vi "MEI.vi"(6 "Numero Stadi":dbl, 7 "TIPO POMPA":u16(ring)=3 items=["ESOB (1450)", "ESOB (2900)", "ESCC (1450)", "ESCC (2900)", "ESCCi (1450)", "ESCCi (2900)", "MS-V (2900)", "MSS (2900)"], 10 "INDEX":T1, 11 "Curva":string[][](array[string])) -> (0 "TIPO POMPA 2":u16(ring)=3 items=["ESOB (1450)", "ESOB (2900)", "ESCC (1450)", "ESCC (2900)", "ESCCi (1450)", "ESCCi (2900)", "MS-V (2900)", "MSS (2900)"], 1 "Numero Stadi 2":dbl, 2 "MEI":string, 3 "colonna mei":string[](array[string]), 5 "annulla ?":bool)   [LabVIEW 2016]
uses:
  TypeDef/Indici.ctl
  <vilib>/Analysis/6fits.llb/Curve Fitting Criteria.ctl
  <vilib>/Analysis/polynomials.llb/nth Derivative of Polynomial (DBL).vi
  <vilib>/Analysis/polynomials.llb/Polynomial Roots (DBL).vi
  <vilib>/Analysis/polynomials.llb/Polynomial Plot (Range).vi
  <vilib>/Analysis/polynomials.llb/Scalar Polynomial Evaluation (DBL).vi
  <vilib>/Analysis/NI_AALPro.lvlib
panel:
  in  "annulla":bool
  out "NewVal":u16
  in  "reinizializza tabella":bool
  in  "elimina acq":bool
  out "Q_PL [l/min]":dbl
  out "Q_OL [l/min]":dbl
  out "Q_BEP [l/min]":dbl
  out "R-square 2":dbl caption="R-square"
  out "R-square":dbl
  in  "AUTOSCALA Q-H":bool=TRUE
  in  "AUTOSCALA Q-ETA":bool=TRUE
  in  "OK Button":bool
  in  "polynomial order Q-H":i32=4
  in  "polynomial order Q-Etap":i32=4
  in  "Test data":i32(listbox)
  out "indice":i32
  out "C_MEI":dbl
  out "C_OL":dbl
  out "C_PL":dbl
  out "C_BEP":dbl
  out "F_Eta":dbl
  out "n_S":dbl
  out "Velocità Nominale":dbl
  out "H_BEP [m]":dbl
  out "Q-H":cluster{"Ramp Pattern":dbl[], "P(A)":dbl[]}[](graph)
  out "ETA_PL [%]":dbl
  out "ETA_OL [%]":dbl
  out "Q_PL [m3/h]":dbl
  out "Q_OL [m3/h]":dbl
  out "ETA_BEP [%]":dbl
  out "Q-ETAp":cluster{"Ramp Pattern":dbl[], "P(A)":dbl[]}[](graph)
  out "Q_BEP [m3/h]":dbl
  # "CALCOLO INDICE MEI"
  # "Selezionare tipologia pompa e numero stadi"
  # "Seleziona ordine delle polinomiali"
  # "Risultati calcoli intermedi"
  # "RISULTATO"
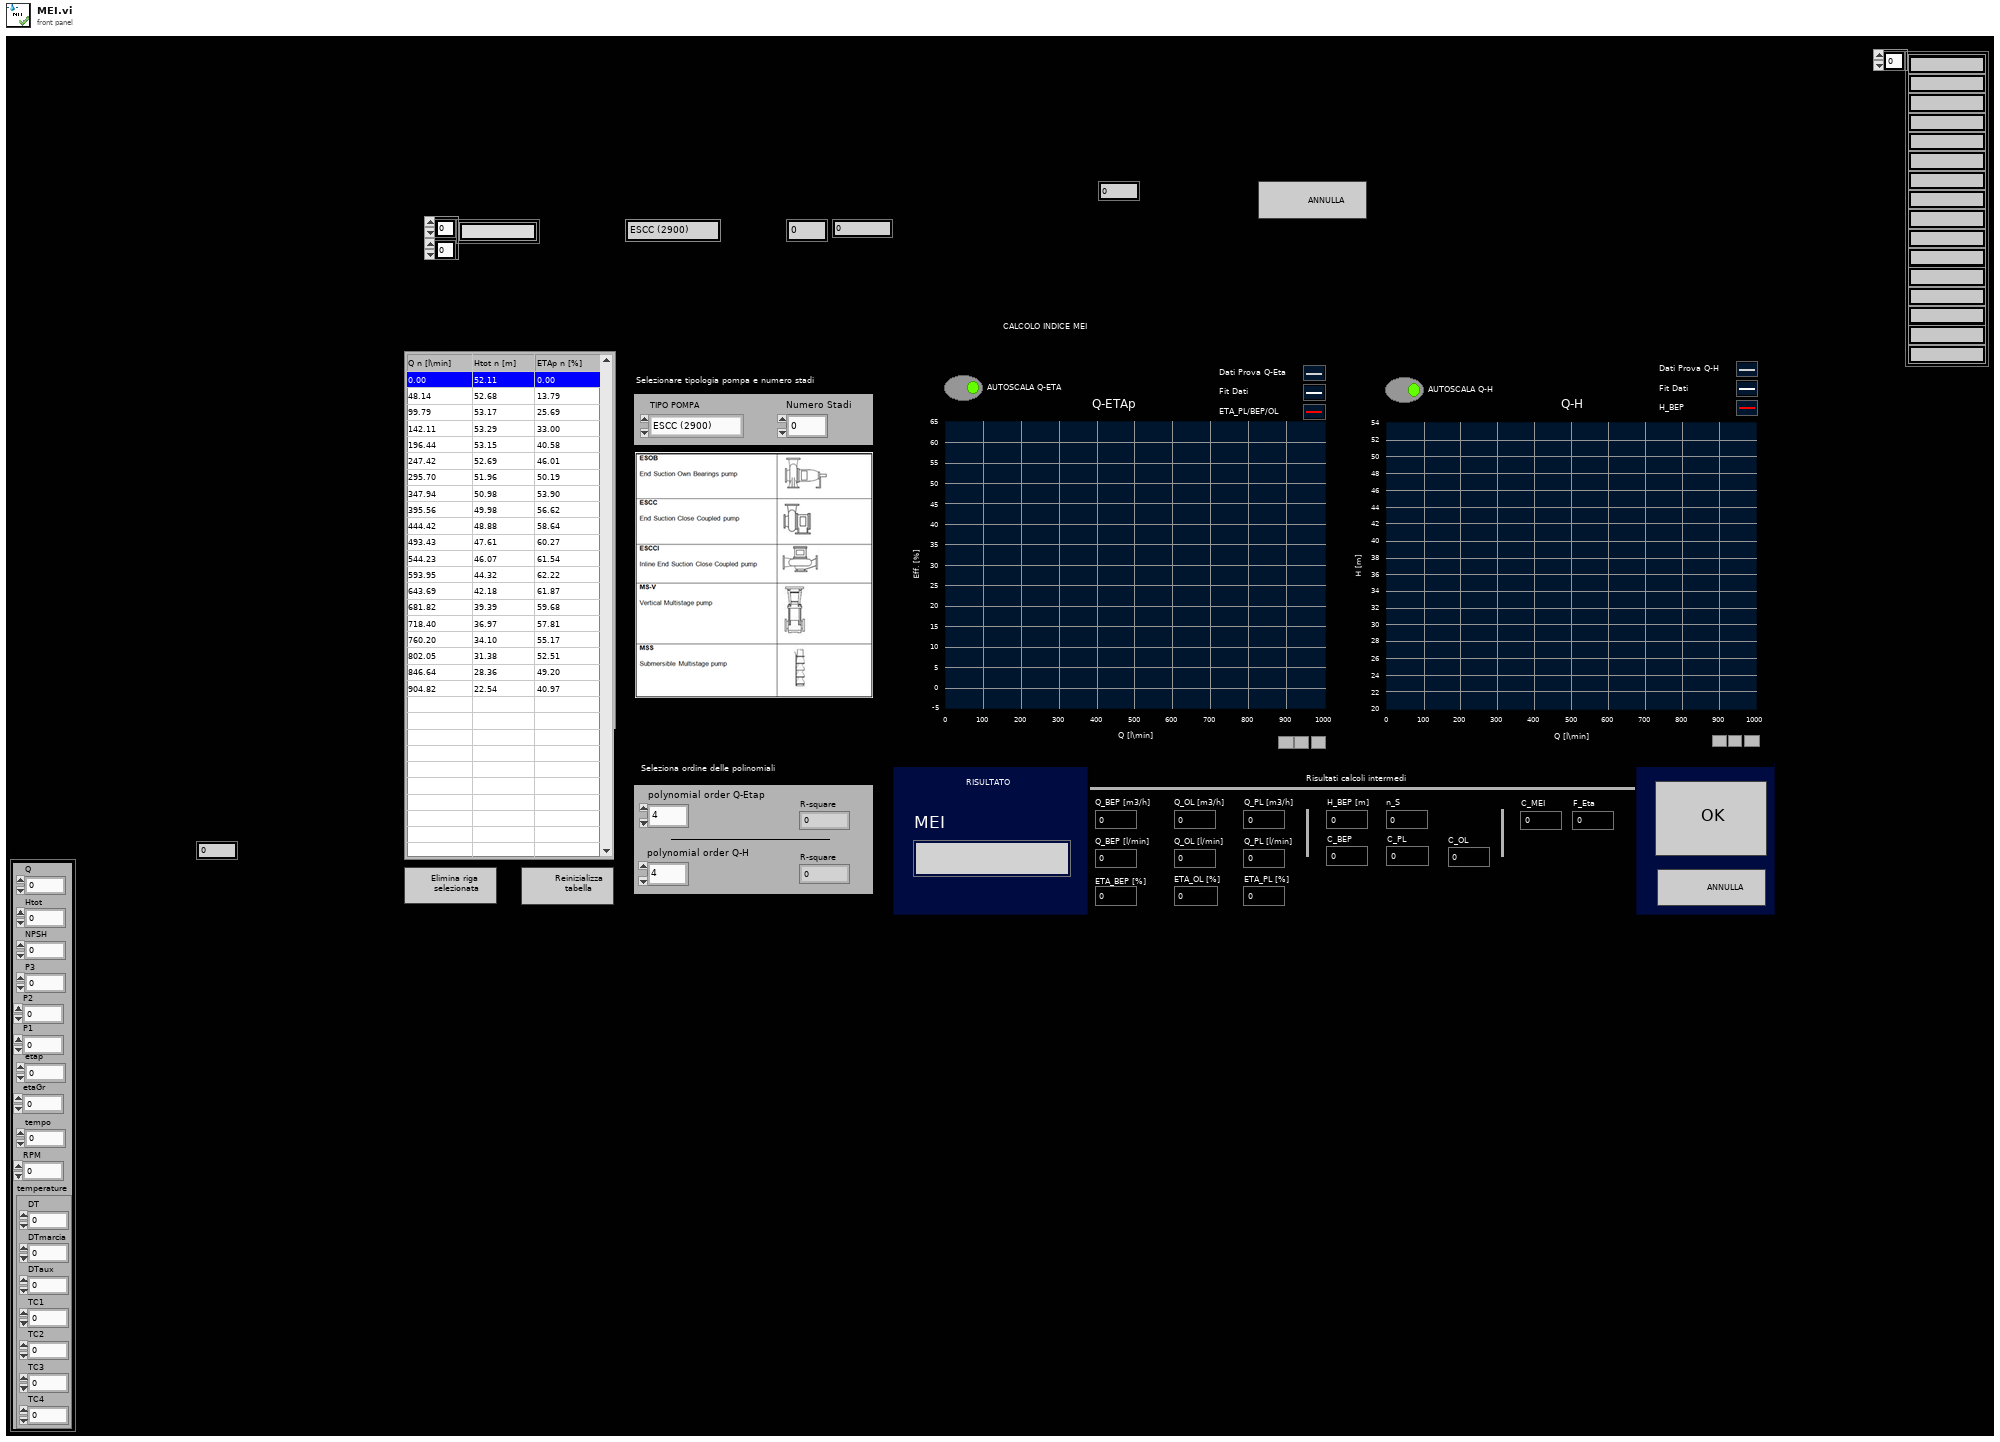
[diagram p1: front panel]
types:
  T1 = typedef "Indici.ctl" = cluster{"Q":i32, "Htot":i32, "NPSH":i32, "P3":i32, "etap":i32, "temperature":cluster{"DT":i32, "DTmarcia":i32, "DTaux":i32, "TC1":i32, "TC2":i32, "TC3":i32, "TC4":i32}, "tempo":i32, "P2":i32, "P1":i32, "etaGr":i32, "RPM":i32}
  T2 = typedef "NI_AALPro.lvlib/Curve Fitting Criteria.ctl" = u16
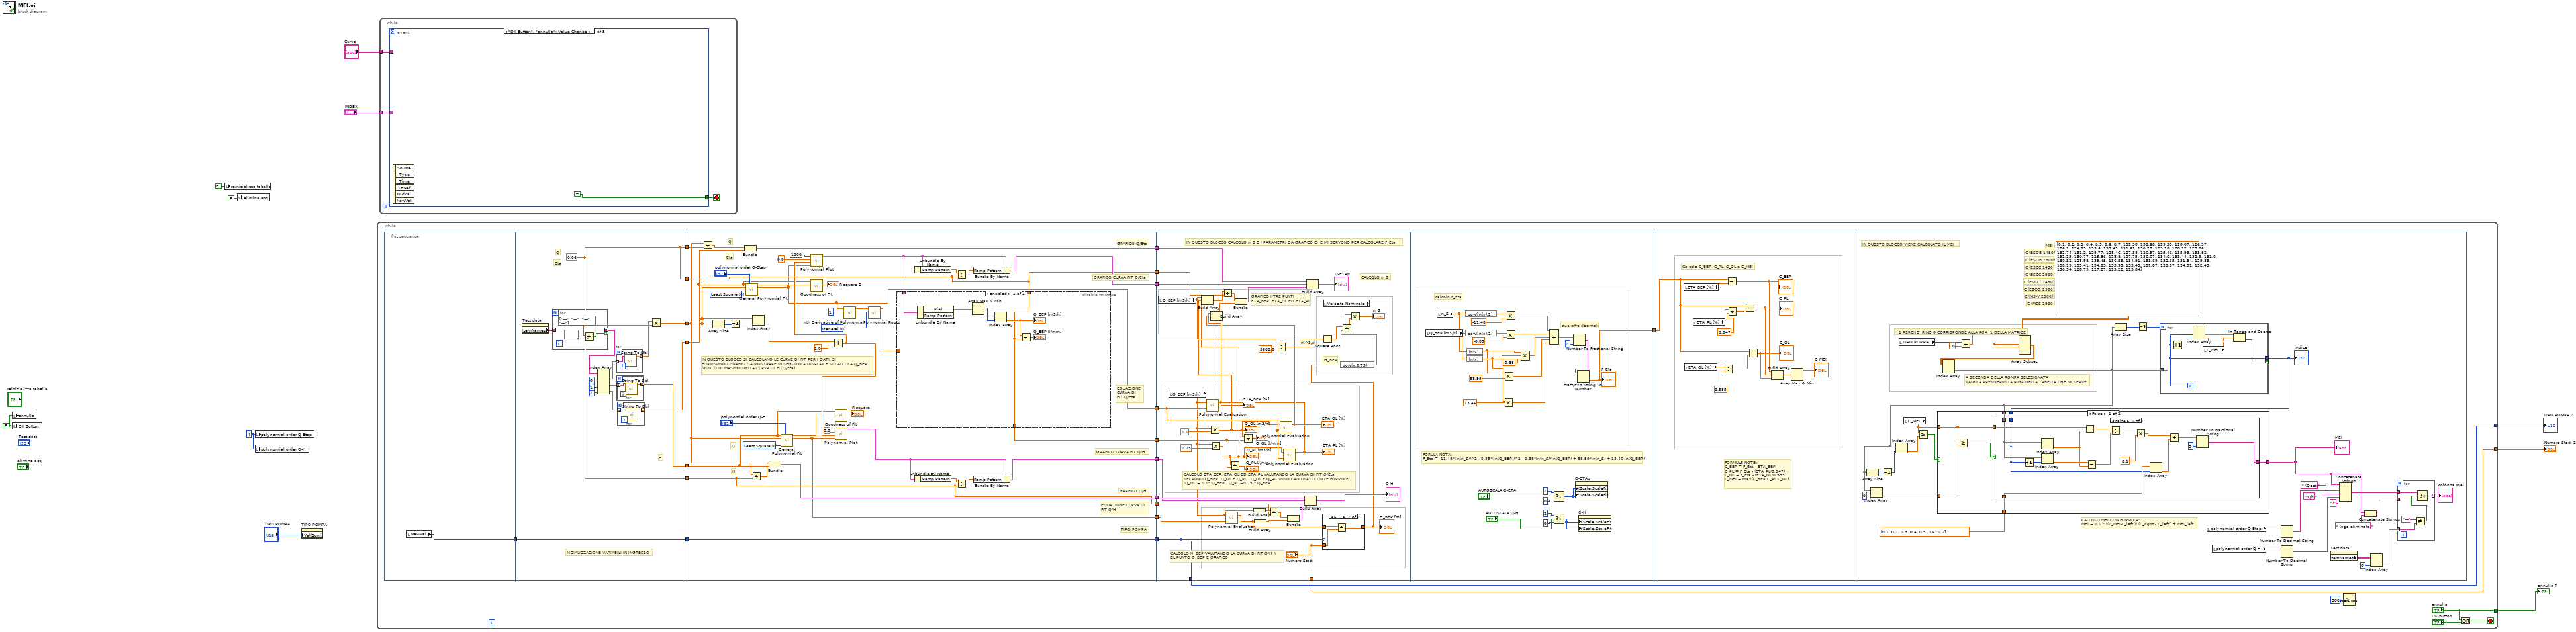
[diagram p0: block diagram]
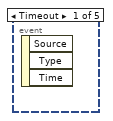
[diagram p2: hidden frame]
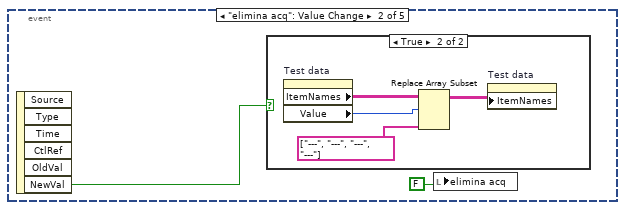
[diagram p3: hidden frame]
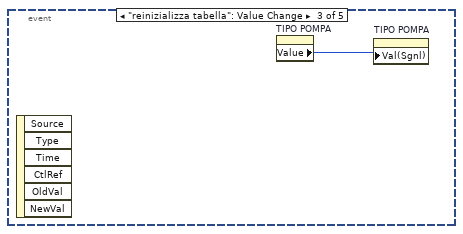
[diagram p5: hidden frame]
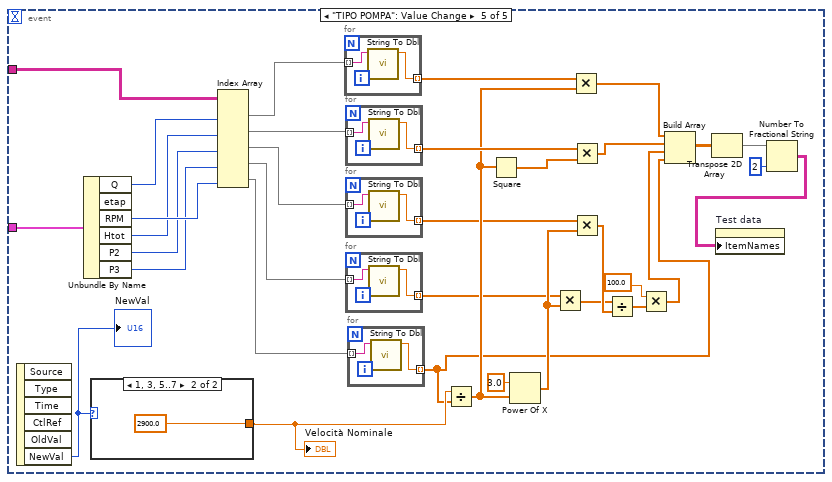
[diagram p6: hidden frame]
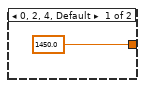
[diagram p7: hidden frame]
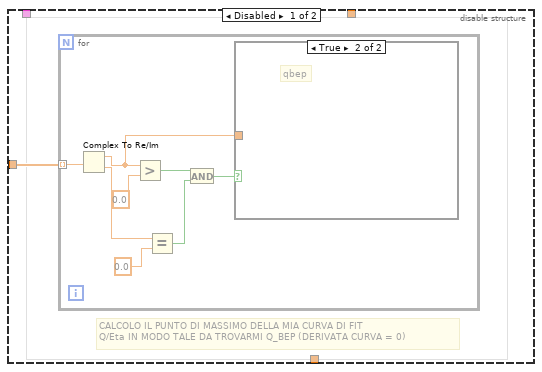
[diagram p8: hidden frame]
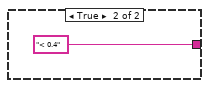
[diagram p11: hidden frame]
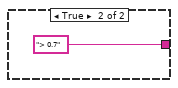
[diagram p12: hidden frame]
diagram:
  w1 = 4 ("polynomial order Q-Etap")
  w3 = FALSE ("OK Button")
  n1 = local write "annulla"(w3) -> ()
  n2 = local write "OK Button"(w3) -> ()
  n3 = local write "reinizializza tabella"(FALSE ("reinizializza tabella")) -> ()
  n4 = local write "elimina acq"(FALSE ("elimina acq")) -> ()
  n5 = local write "polynomial order Q-Etap"(w1) -> ()
  n6 = local write "polynomial order Q-H"(w1) -> ()
  n7 = property on="TIPO POMPA" class="Ring (strict)"("Val(Sgnl)"="TIPO POMPA") -> ()  [unwired: 2 in, 2 out]
  n8 = while {
    tunnel: [w22] -> w10
    tunnel: [w21] -> w9
    tunnel: ["annulla"] -> w2
    stop <- w12 stop-if-true
    n9 = flat-sequence {
      tunnel: [w36] -> w13
      tunnel: [w50] -> w35
      tunnel: [w42] -> w34
      tunnel: [w37] -> w33
      tunnel: [w49] -> w20
      tunnel: [w49] -> w19
      tunnel: [w49] -> w18
      tunnel: [w40] -> w14
      tunnel: w13 -> [w37]
      tunnel: [w93] -> w32
      tunnel: [w67] -> w31
      tunnel: [w75] -> w30
      tunnel: [w92] -> w29
      tunnel: [w63] -> w28
      tunnel: [w88] -> w27
      tunnel: w35 -> [w72]
      tunnel: w34 -> [w80]
      tunnel: [w87] -> w26
      tunnel: w33 -> [w87]
      tunnel: w20 -> [w73]
      tunnel: w19 -> [w62]
      tunnel: w18 -> [w61]
      tunnel: [w61] -> w17
      tunnel: [w62] -> w16
      tunnel: [w60] -> w15
      tunnel: w14 -> [w77]
      tunnel: w32 -> [w139]
      tunnel: w31 -> [w138]
      tunnel: w30 -> [w155]
      tunnel: w29 -> [w153]
      tunnel: w28 -> [w152]
      tunnel: w27 -> [w147]
      tunnel: w26 -> [w132]
      tunnel: [w132] -> w22
      tunnel: ["Numero Stadi"] -> w21
      tunnel: w17 -> [w128]
      tunnel: w16 -> [w125]
      tunnel: w15 -> [w121]
      tunnel: [w187] -> w25
      tunnel: w25 -> [w198]
      frame #0 {
        n10 = local read "NewVal"() -> (w36:u16)
      }
      frame #1 {
        w49 = 0.06
        # "NIZIALIZZAZIONE VARIABILI IN INGRESSO"
        # "Eta"
        # "H"
        # "Q"
        n11 = property on="Test data" class="MCListbox (strict)"() -> ("ItemNames"=w39:string[][])  [unwired: 2 in, 2 out]
        n12 = for {
          tunnel: w39 -> [w52] mode=indexing
          tunnel: [w52] -> w38 mode=indexing if=w51
          n13 = Not Equal?(x=string[] ["---", "---", "---", "---"] ("new element/subarray"), y=w52) -> (x != y?=w51:bool)
        }
        n14 = Index Array(array=w38, index (col) #1=0 ("disabled index (col)"), index (col) #2=1 ("index (col)"), index (col) #3=2 ("index (col)")) -> (element #1=w45:string[], element #2=w43:string[], element #3=w41:string[])  [unwired: 3 in]
        n15 = for {
          tunnel: w45 -> [w59] mode=indexing
          tunnel: [w58] -> w44 mode=indexing
          n16 = call "String To Dbl.vi"("String"=w59) -> ("Numeric"=w58:dbl)  [unwired: 10 in]
        }
        n17 = for {
          tunnel: w43 -> [w57] mode=indexing
          tunnel: [w56] -> w42 mode=indexing
          n18 = call "String To Dbl.vi"("String"=w57) -> ("Numeric"=w56:dbl)  [unwired: 10 in]
        }
        n19 = for {
          tunnel: w41 -> [w55] mode=indexing
          tunnel: [w54] -> w40 mode=indexing
          n20 = call "String To Dbl.vi"("String"=w55) -> ("Numeric"=w54:dbl)  [unwired: 10 in]
        }
        n21 = Multiply(x=w44, y=w49) -> (x*y=w50:dbl[])
      }
      frame #2 {
        w90 = T2 0 items=["Least Square", "Least Absolute Residual", "Bisquare"] ("method")
        w97 = u16 0 items=["General", "Simple Classification", "Refinement", "Advanced Refinement"] ("option")
        w101 = T2 0 items=["Least Square", "Least Absolute Residual", "Bisquare"] ("method")
        # "TIPO POMPA"
        # "IN QUESTO BLOCCO SI CALCOLANO LE CURVE DI FIT PER I DATI, SI \nFORNISONO I GRAFICI DA MOSTRARE IN SEGUITO A DISPLAY E SI CALCOLA Q_BEP \n(PUNTO DI MASIMO DELLA CURVA DI FITQ/Eta)"
        # "H"
        # "Q"
        # "EQUAZIONE CURVA DI \nFIT Q/H"
        # "EQUAZIONE \nCURVA DI \nFIT Q/Eta"
        # "GRAFICO CURVA FIT Q/H"
        # "GRAFICO Q/H"
        # "GRAFICO CURVA FIT Q/Eta"
        # "GRAFICO Q/Eta"
        # "Q"
        # "Eta"
        n22 = Divide(x=w72, y=w73) -> (x/y=w74:dbl[])
        n23 = Array Size(array=w72) -> (size(s)=w86:i32)
        n24 = Decrement(x=w86) -> (x-1=w85:i32)
        n25 = Bundle(w74, w77) -> (w93:cluster{dbl[], dbl[]})  [unwired: 1 in]
        n26 = call <vilib>:"General Polynomial Fit.vi"("Y"=w77, "polynomial order"="polynomial order Q-Etap", "X"=w72, "method"=w101) -> ("Best Polynomial Fit"=w76:dbl[], "Polynomial Coefficients"=w75:dbl[])  [unwired: 8 in, 2 out]
        n27 = Divide(x=w72, y=w62) -> (x/y=w71:dbl[])
        n28 = Index Array(array=w72, index=w85) -> (element=w84:dbl)
        n29 = Bundle(w71, w80) -> (w92:cluster{dbl[], dbl[]})  [unwired: 1 in]
        n30 = call <vilib>:"General Polynomial Fit.vi"("Y"=w80, "polynomial order"="polynomial order Q-H", "X"=w72, "method"=w90) -> ("Best Polynomial Fit"=w81:dbl[], "Polynomial Coefficients"=w88:dbl[])  [unwired: 8 in, 2 out]
        n31 = call <vilib>:"Goodness of Fit.vi"("Best Fit"=w76, "Y"=w77) -> ("R-square"=→"R-square 2":dbl)  [unwired: 6 in, 3 out]
        n32 = Add(x=w84, y=1.0) -> (x+y=w82:dbl)
        n33 = call-poly <vilib>:"Polynomial Plot.vi"("P(x)"=w75, "end"=w82, "start"=0.0, "samples"=1000) -> ("polynomial plot"=w68:cluster{"Ramp Pattern":dbl[], "P(A)":dbl[]})  [unwired: 6 in, 1 out]
        n34 = call <vilib>:"Goodness of Fit.vi"("Best Fit"=w81, "Y"=w80) -> ("R-square"=→"R-square":dbl)  [unwired: 6 in, 3 out]
        n35 = call-poly <vilib>:"Polynomial Plot.vi"("P(x)"=w88, "end"=w82, "start"=0.0) -> ("polynomial plot"=w64:cluster{"Ramp Pattern":dbl[], "P(A)":dbl[]})  [unwired: 7 in, 1 out]
        n36 = call-poly <vilib>:"nth Derivative of Polynomial.vi"("order"=1, "P(x)"=w75) -> ("Nth Derivative of P(x)"=w98:dbl[])  [unwired: 8 in, 1 out]
        n37 = call-poly <vilib>:"Polynomial Roots.vi"("option"=w97, "P(x)"=w98) -> ("Roots"=w96:cdb[])  [unwired: 8 in, 1 out]
        n38 = disable-structure shown="Enabled" {
          disable-tunnel: w96 -> [w102 _]
          disable-tunnel: w68 -> [_ w117]
          disable-tunnel: w61 -> [_ w111]
          disable-tunnel: [_ w111] -> w60
          frame Disabled {
            # "CALCOLO IL PUNTO DI MASSIMO DELLA MIA CURVA DI FIT\nQ/Eta IN MODO TALE DA TROVARMI Q_BEP (DERIVATA CURVA = 0)"
            n39 = for {
              tunnel: w102 -> [w109] mode=indexing
              n40 = Complex To Re/Im(x + iy=w109) -> (x=w108:dbl, y=w104:dbl)
              n41 = Greater?(x=w108, y=0.0) -> (0:w107:bool)
              n42 = Equal?(x=w104, y=0.0) -> (x = y?=w106:bool)
              n43 = And(x=w107, y=w106) -> (x .and. y?=w105:bool)
              n44 = case shown="True" w105 {
                tunnel: w108 -> [_ _]
                frame False {
                }
                frame True {
                  # "qbep"
                }
              }
            }
          }
          frame Enabled {
            n45 = Unbundle By Name(w117) -> ("P(A)"=w116:dbl[], "Ramp Pattern"=w114:dbl[])
            n46 = Array Max & Min(array=w116) -> (max index (indices)=w115:i32)  [unwired: 3 out]
            n47 = Index Array(array=w114, index=w115) -> (element=w112:dbl)
            "Q_BEP [m3/h]" <- w112
            n48 = Divide(x=w112, y=w111) -> (x/y=→"Q_BEP [l/min]":dbl)
          }
        }
        n49 = Unbundle By Name(w68) -> ("Ramp Pattern"=w70:dbl[])
        n50 = Unbundle By Name(w64) -> ("Ramp Pattern"=w65:dbl[])
        n51 = Divide(x=w70, y=w61) -> (x/y=w69:dbl[])
        n52 = Divide(x=w65, y=w62) -> (x/y=w66:dbl[])
        n53 = Bundle By Name(cluster=w68, "Ramp Pattern"=w69) -> (w67:cluster{"Ramp Pattern":dbl[], "P(A)":dbl[]})
        n54 = Bundle By Name(cluster=w64, "Ramp Pattern"=w66) -> (w63:cluster{"Ramp Pattern":dbl[], "P(A)":dbl[]})
      }
      frame #3 {
        # "m^3/s"
        # "CALCOLO H_BEP VALUTANDO LA CURVA DI FIT Q/H N\nEL PUNTO Q_BEP E GRAFICO"
        # "CALCOLO ETA_BEP, ETA_OL ED ETA_PL VALUTANDO LA CURVA DI FIT Q/Eta \nNEI PUNTI Q_BEP, Q_OL E Q_PL.  Q_OL E Q_PL SONO CALCOLATI CON LE FORMULE\n Q_OL = 1.1* Q_BEP , Q_PL =0.75 * Q_BEP"
        # "GRAFICO I TRE PUNTI\nETA_BEP, ETA_OL ED ETA_PL"
        # "H_BEP"
        # "CALCOLO n_S"
        # "IN QUESTO BLOCCO CALCOLO n_S E I PARAMETRI DA GRAFICO CHE MI SERVONO PER CALCOLARE F_Eta"
        n55 = local read "Q_BEP [m3/h]"() -> (w135:dbl)
        n56 = local read "Q_BEP [m3/h]"() -> (w146:dbl)
        n57 = call-poly <vilib>:"Polynomial Evaluation.vi"("P(x)"=w155, "a"=w146) -> ("P(a)"=w151:dbl)  [unwired: 1 out]
        "ETA_BEP [%]" <- w151
        n58 = Multiply(x=w146, y=1.1) -> (x*y=w124:dbl)
        "Q_OL [m3/h]" <- w124
        n59 = Multiply(x=w146, y=0.75) -> (x*y=w122:dbl)
        "Q_PL [m3/h]" <- w122
        n60 = Build Array(w135, w124, w122) -> (w130:dbl[])
        n61 = Divide(x=w130, y=w128) -> (x/y=w129:dbl[])
        n62 = call-poly <vilib>:"Polynomial Evaluation.vi"("P(x)"=w147, "a"=w146) -> ("P(a)"=w133:dbl)  [unwired: 1 out]
        n63 = Divide(x=w122, y=w121) -> (x/y=→"Q_PL [l/min]":dbl)
        n64 = Divide(x=w124, y=w121) -> (x/y=→"Q_OL [l/min]":dbl)
        n65 = Build Array(w146) -> (w126:dbl[])
        n66 = Build Array(w133) -> (w145:dbl[])
        n67 = Divide(x=w126, y=w125) -> (x/y=w127:dbl[])
        n68 = Divide(x=w135, y=3600.0) -> (x/y=w134:dbl)
        n69 = call-poly <vilib>:"Polynomial Evaluation.vi"("P(x)"=w155, "a"=w124) -> ("P(a)"=w150:dbl)  [unwired: 1 out]
        "ETA_OL [%]" <- w150
        n70 = call-poly <vilib>:"Polynomial Evaluation.vi"("P(x)"=w155, "a"=w122) -> ("P(a)"=w149:dbl)  [unwired: 1 out]
        "ETA_PL [%]" <- w149
        n71 = Build Array(w151, w150, w149) -> (w148:dbl[])
        n72 = Bundle(w129, w148) -> (w119:cluster{dbl[], dbl[]})  [unwired: 1 in]
        n73 = Bundle(w127, w145) -> (w118:cluster{dbl[], dbl[]})  [unwired: 1 in]
        n74 = Build Array(w153, w152, w118) -> (→"Q-H":cluster{"Ramp Pattern":dbl[], "P(A)":dbl[]}[])
        n75 = Build Array(w139, w138, w119) -> (→"Q-ETAp":cluster{"Ramp Pattern":dbl[], "P(A)":dbl[]}[])
        n76 = Square Root(x=w134) -> (sqrt(x)=w144:dbl)
        n77 = case shown="6, 7" w132 {
          tunnel: [w159 w162] -> w140
          tunnel: w133 -> [w159 w161]
          tunnel: "Numero Stadi" -> [_ w160]
          frame 0, Default {
          }
          frame 6, 7 {
            n78 = Divide(x=w161, y=w160) -> (x/y=w162:dbl)
          }
        }
        "H_BEP [m]" <- w140
        n79 = local read "Velocità Nominale"() -> (w141:dbl)
        n80 = expression code="pow(x,0.75)"(w140) -> (w137:dbl)
        n81 = Divide(x=w144, y=w137) -> (x/y=w143:dbl)
        n82 = Multiply(x=w141, y=w143) -> (x*y=→"n_S":dbl)
      }
      frame #4 {
        # "FORULA NOTA:\nF_Eta = -11.48*(ln(n_S))^2 - 0.85*(ln(Q_BEP))^2 - 0.38*ln(n_S)*ln(Q_BEP) + 88.59*ln(n_S) + 13.46 ln(Q_BEP)"
        # "due cifre decimali"
        # "calcolo F_Eta"
        n83 = local read "Q_BEP [m3/h]"() -> (w174:dbl)
        n84 = local read "n_S"() -> (w178:dbl)
        n85 = expression code="pow(ln(x),2)"(w178) -> (w186:dbl)
        n86 = expression code="pow(ln(x),2)"(w174) -> (w184:dbl)
        n87 = expression code="ln(x)"(w178) -> (w171:dbl)
        n88 = expression code="ln(x)"(w174) -> (w172:dbl)
        n89 = Multiply(x=w172, y=13.46) -> (x*y=w173:dbl)
        n90 = Multiply(x=w171, y=88.59) -> (x*y=w176:dbl)
        n91 = Multiply(x=w186, y=-11.48) -> (x*y=w182:dbl)
        n92 = Multiply(x=w184, y=-0.85) -> (x*y=w181:dbl)
        n93 = Compound Arithmetic op=MULTIPLY(w171, w172, -0.38 ("value")) -> (w179:dbl)
        n94 = Compound Arithmetic op=ADD(w182, w181, w179, w176, w173) -> (w190:dbl)
        n95 = Select(t=u8 2 ("X Scale.Scale Fit"), s="AUTOSCALA Q-ETA", f=u8 0 ("X Scale.Scale Fit")) -> (s? t:f=w163:u8)
        n96 = Select(t=u8 2 ("X Scale.Scale Fit"), s="AUTOSCALA Q-H", f=u8 0 ("X Scale.Scale Fit")) -> (s? t:f=w164:u8)
        n97 = Number To Fractional String(number=w190, precision (6)=i16 2) -> (F-format string=w188:string)  [unwired: 2 in]
        n98 = property on="Q-ETAp" class="XYGraph (strict)"("XScale.ScaleFit"=w163, "YScale.ScaleFit"=w163) -> ()  [unwired: 2 in, 2 out]
        n99 = Fract/Exp String To Number(string=w188) -> (number=w187:dbl)  [unwired: 3 in, 1 out]
        "F_Eta" <- w187
        n100 = property on="Q-H" class="XYGraph (strict)"("XScale.ScaleFit"=w164, "YScale.ScaleFit"=w164) -> ()  [unwired: 2 in, 2 out]
      }
      frame #5 {
        # "FORMULE NOTE:\nC_BEP = F_Eta - ETA_BEP\nC_PL = F_Eta - (ETA_PL/0.947)\nC_OL = F_Eta - (ETA_OL/0.985)\nC_MEI = max(C_BEP,C_PL,C_OL)"
        # "Calcolo C_BEP, C_PL, C_OL e C_MEI"
        n101 = local read "ETA_BEP [%]"() -> (w203:dbl)
        n102 = local read "ETA_OL [%]"() -> (w197:dbl)
        n103 = local read "ETA_PL [%]"() -> (w201:dbl)
        n104 = Divide(x=w197, y=0.985) -> (x/y=w196:dbl)
        n105 = Subtract(x=w198, y=w203) -> (x-y=w195:dbl)
        "C_BEP" <- w195
        n106 = Divide(x=w201, y=0.947) -> (x/y=w200:dbl)
        n107 = Subtract(x=w198, y=w200) -> (x-y=w194:dbl)
        "C_PL" <- w194
        n108 = Subtract(x=w198, y=w196) -> (x-y=w193:dbl)
        "C_OL" <- w193
        n109 = Build Array(w195, w194, w193) -> (w192:dbl[])
        n110 = Array Max & Min(array=w192) -> (max value=→"C_MEI":dbl)  [unwired: 3 out]
      }
      frame #6 {
        # "CALCOLO MEI CON FORMULA:\nMEI = 0.1 * ((C_MEI-C_left )/ (C_right - C_left)) + MEI_left"
        # "+1 PERCHE' RING 0 CORRISPONDE ALLA RGA  1 DELLA MATRICE"
        # "A SECONDA DELLA POMPA SELEZIONATA\nVADO A PRENDERMI LA RIGA DELLA TABELLA CHE MI SERVE"
        # "IN QUESTO BLOCCO VIENE CALCOLATO IL MEI"
        # "C (MSS 2900)"
        # "C (MS-V 2900)"
        # "C (ESCCi 2900)"
        # "C (ESCCi 1450)"
        # "C (ESCC 2900)"
        # "C (ESCC 1450)"
        # "C (ESOB 2900)"
        # "C (ESOB 1450)"
        # "MEI"
        n111 = local read "TIPO POMPA"() -> (w233:u16)
        n112 = local read "C_MEI"() -> (w224:dbl)
        n113 = Add(x=w233, y=1.0) -> (x+y=w232:dbl)
        n114 = Array Subset(array=dbl[][] [[0.1, 0.2, 0.3, 0.4, 0.5, 0.6, 0.7], [132.58, 130.68, 129.35, 128.07, 126.97, 126.1, 124.85], [135.6, 133.43, 131.61, 130.27, 129.18, 128.12, 127.06], [132.74, 131.2, 129.77, 128.46, 127.38, 126.57, 125.46], [135.93, 133.82, 132.23, 130.77, 129.86, 128.8, 127.75], [136.67, 134.6, 133.44, 132.3, 131.0, 130.32, 128.98], [139.45, 136.53, 134.91, 133.69, 132.65, 131.34, 129.83], [138.19, 135.41, 134.89, 133.95, 133.43, 131.87, 130.37], [134.31, 132.43, 130.94, 128.79, 127.27, 125.22, 123.84]], index (row)=w232, length (row)=w232) -> (w234:dbl[][])  [unwired: 2 in]
        n115 = Index Array(array=w234) -> (element=w220:dbl[])  [unwired: 2 in]
        n116 = Array Size(array=w220) -> (size(s)=w228:i32)
        n117 = Index Array(array=w220, index=0) -> (element=w222:dbl)
        n118 = Decrement(x=w228) -> (x-1=w227:i32)
        n119 = Index Array(array=w220, index=w227) -> (element=w226:dbl)
        n120 = Less Or Equal?(x=w224, y=w226) -> (x <= y?=w225:bool)
        n121 = Array Size(array=w220) -> (size(s)=w230:i32)
        n122 = Decrement(x=w230) -> (x-1=w229:i32)
        n123 = for {
          N: w229 -> [_]
          tunnel: w220 -> [w272]
          tunnel: [w268] -> w219 if=w267
          tunnel: [w267] -> _ mode=indexing
          i -> [w268]
          n124 = Increment(x=w268) -> (x+1=w273:i32)
          n125 = Index Array(array=w272, index #1=w268, index #2=w273) -> (element #1=w271:dbl, element #2=w270:dbl)
          n126 = local read "C_MEI"() -> (w269:dbl)
          n127 = In Range and Coerce(upper limit=w271, x=w269, lower limit=w270) -> (In Range?=w267:bool)  [unwired: 1 out]
        }
        "indice" <- w219
        n128 = case shown="False" w225 {
          tunnel: [w246 "> 0.7"] -> w205
          tunnel: w224 -> [w245 _]
          tunnel: w222 -> [w248 _]
          tunnel: w219 -> [w244 _]
          tunnel: dbl[] [0.1, 0.2, 0.3, 0.4, 0.5, 0.6, 0.7] -> [w243 _]
          tunnel: w220 -> [w242 _]
          frame False {
            n129 = Greater Or Equal?(x=w245, y=w248) -> (x >= y?=w247:bool)
            n130 = case shown="False" w247 {
              tunnel: [w253 "< 0.4"] -> w246
              tunnel: w245 -> [w264 _]
              tunnel: w244 -> [w250 _]
              tunnel: w243 -> [w251 _]
              tunnel: w242 -> [w252 _]
              frame False {
                n131 = Increment(x=w250) -> (x+1=w263:i32)
                n132 = Index Array(array=w252, index=w263) -> (element=w262:dbl)
                n133 = Index Array(array=w252, index=w250) -> (element=w256:dbl)
                n134 = Subtract(x=w264, y=w256) -> (x-y=w261:dbl)
                n135 = Subtract(x=w262, y=w256) -> (x-y=w260:dbl)
                n136 = Divide(x=w261, y=w260) -> (x/y=w259:dbl)
                n137 = Multiply(x=w259, y=0.1 ("C_MEI")) -> (x*y=w257:dbl)
                n138 = Index Array(array=w251, index=w250) -> (element=w249:dbl)
                n139 = Add(x=w257, y=w249) -> (x+y=w255:dbl)
                n140 = Number To Fractional String(number=w255, precision (6)=i16 2) -> (F-format string=w253:string)  [unwired: 2 in]
              }
              frame True {
              }
            }
          }
          frame True {
          }
        }
        "MEI" <- w205
        n141 = local read "polynomial order Q-Etap"() -> (w216:i32)
        n142 = local read "polynomial order Q-H"() -> (w215:i32)
        n143 = Number To Decimal String(number=w216) -> (decimal integer string=w214:string)  [unwired: 1 in]
        n144 = Number To Decimal String(number=w215) -> (decimal integer string=w213:string)  [unwired: 1 in]
        n145 = property on="Test data" class="MCListbox (strict)"() -> ("ItemNames"=w211:string[][])  [unwired: 2 in, 2 out]
        n146 = Concatenate Strings(w205, " (Qeta:" ("string"), w214, ";Qh:" ("string"), w213, ")" ("string")) -> (w208:string)
        n147 = Concatenate Strings(w205, " (riga eliminata)" ("string")) -> (w204:string)
        n148 = Index Array(array=w211, index (col)=0 ("disabled index (col)")) -> (element=w209:string[])  [unwired: 1 in]
        n149 = for {
          tunnel: w209 -> [w241] mode=indexing
          tunnel: w208 -> [w239]
          tunnel: [w237] -> w207 mode=indexing
          tunnel: w204 -> [w236]
          n150 = Not Equal?(x="---", y=w241) -> (x != y?=w240:bool)
          n151 = Select(t=w239, s=w240, f=w236) -> (s? t:f=w237:string)
        }
        "colonna mei" <- w207
      }
    }
    n152 = Wait (ms)(milliseconds to wait=u32 500) -> ()  [unwired: 1 out]
    n153 = Or(x="annulla", y="OK Button") -> (x .or. y?=w12:bool)
  }
  "TIPO POMPA 2" <- w10
  "Numero Stadi 2" <- w9
  "annulla ?" <- w2
  n154 = while {
    tunnel: "INDEX" -> [w275]
    tunnel: "Curva" -> [w274]
    stop <- w276 stop-if-true
    n155 = event shown="[3] \"OK Button\", \"annulla\": Value Change" {
      selector: _ -> [_ _ _ _ _]
      dyn-events: _ -> [_ _ _ _ _]
      timeout: _ -> [_ _ _ _ _]
      tunnel: [_ _ _ TRUE _] -> w276
      tunnel: w275 -> [_ _ _ _ w290]
      tunnel: w274 -> [_ _ _ _ w289]
      event Timeout {
        n156 = event-data() -> ()  [unwired: 1 in, 3 out]
      }
      event "elimina acq": Value Change {
        n157 = event-data() -> ("NewVal"=w278:bool)  [unwired: 1 in, 5 out]
        n158 = case shown="True" w278 {
          frame False {
          }
          frame True {
            n159 = property on="Test data" class="MCListbox (strict)"() -> ("ItemNames"=w282:string[][], "Value"=w280:i32)  [unwired: 2 in, 2 out]
            n160 = Replace Array Subset(array=w282, new element=string[] ["---", "---", "---", "---"] ("new element/subarray"), index (row)=w280) -> (w281:string[][])  [unwired: 1 in]
            n161 = property on="Test data" class="MCListbox (strict)"("ItemNames"=w281) -> ()  [unwired: 2 in, 2 out]
          }
        }
        n162 = local write "elimina acq"(FALSE ("elimina acq")) -> ()
      }
      event "reinizializza tabella": Value Change {
        n163 = event-data() -> ()  [unwired: 1 in, 6 out]
        n164 = property on="TIPO POMPA" class="Ring (strict)"() -> ("Value"=w283:u16)  [unwired: 2 in, 2 out]
        n165 = property on="TIPO POMPA" class="Ring (strict)"("Val(Sgnl)"=w283) -> ()  [unwired: 2 in, 2 out]
      }
      event "OK Button", "annulla": Value Change {
        n166 = event-data() -> ()  [unwired: 1 in, 6 out]
      }
      event "TIPO POMPA": Value Change {
        n167 = event-data() -> ("NewVal"=w291:u16)  [unwired: 1 in, 5 out]
        "NewVal" <- w291
        n168 = Unbundle By Name(w290) -> ("Q"=w303:i32, "RPM"=w307:i32, "Htot"=w304:i32, "P2"=w305:i32, "P3"=w306:i32)  [unwired: 1 out]
        n169 = case shown="1, 3, 5..7" w291 {
          tunnel: [1450.0 ("n_N") 2900.0 ("n_N")] -> w286
          frame 0, 2, 4, Default {
          }
          frame 1, 3, 5..7 {
          }
        }
        "Velocità Nominale" <- w286
        n170 = Index Array(array=w289, index (col) #1=w303, index (col) #2=w304, index (col) #3=w305, index (col) #4=w306, index (col) #5=w307) -> (element #1=w299:string[], element #2=w300:string[], element #3=w301:string[], element #4=w302:string[], element #5=w308:string[])  [unwired: 5 in]
        n171 = for {
          tunnel: w299 -> [w330] mode=indexing
          tunnel: [w329] -> w313 mode=indexing
          n172 = call "String To Dbl.vi"("String"=w330) -> ("Numeric"=w329:dbl)  [unwired: 10 in]
        }
        n173 = for {
          tunnel: w300 -> [w328] mode=indexing
          tunnel: [w327] -> w316 mode=indexing
          n174 = call "String To Dbl.vi"("String"=w328) -> ("Numeric"=w327:dbl)  [unwired: 10 in]
        }
        n175 = for {
          tunnel: w301 -> [w326] mode=indexing
          tunnel: [w325] -> w310 mode=indexing
          n176 = call "String To Dbl.vi"("String"=w326) -> ("Numeric"=w325:dbl)  [unwired: 10 in]
        }
        n177 = for {
          tunnel: w302 -> [w324] mode=indexing
          tunnel: [w323] -> w311 mode=indexing
          n178 = call "String To Dbl.vi"("String"=w324) -> ("Numeric"=w323:dbl)  [unwired: 10 in]
        }
        n179 = for {
          tunnel: w308 -> [w322] mode=indexing
          tunnel: [w321] -> w285 mode=indexing
          n180 = call "String To Dbl.vi"("String"=w322) -> ("Numeric"=w321:dbl)  [unwired: 10 in]
        }
        n181 = Divide(x=w286, y=w285) -> (x/y=w315:dbl[])
        n182 = Square(x=w315) -> (x^2=w314:dbl[])
        n183 = Power Of X(1:w315, 2:3.0 ("x")) -> (0:w312:dbl[])
        n184 = Multiply(x=w311, y=w312) -> (x*y=w317:dbl[])
        n185 = Multiply(x=w313, y=w315) -> (x*y=w295:dbl[])
        n186 = Multiply(x=w316, y=w314) -> (x*y=w294:dbl[])
        n187 = Multiply(x=w310, y=w312) -> (x*y=w318:dbl[])
        n188 = Divide(x=w317, y=w318) -> (x/y=w293:dbl[])
        n189 = Multiply(x=100.0, y=w293) -> (x*y=w288:dbl[])
        n190 = Build Array(w295, w294, w288, w285) -> (w298:dbl[][])
        n191 = Transpose 2D Array(2D array=w298) -> (transposed array=w297:dbl[][])
        n192 = Number To Fractional String(number=w297, precision (6)=i16 2) -> (F-format string=w292:string[][])  [unwired: 2 in]
        n193 = property on="Test data" class="MCListbox (strict)"("ItemNames"=w292) -> ()  [unwired: 2 in, 2 out]
      }
    }
  }
